vi "Generate Non Text Layer(s).vi"(0 "Library Path":path, 5 "new picture":picture, 7 "VI Refnum in":refnum<vi>, 11 "error in":errorcluster) -> (4 "Layers":refnum<class "Layer.lvclass">[](array[class]), 6 "Icon Height":i16, 15 "error out":errorcluster)   [LabVIEW 2024, in "Text-Based VI Icon.lvlib"]
uses:
  <vilib>/LabVIEW Icon API/Set Text Icon/Text-Based VI Icon.lvlib
  <vilib>/LabVIEW Icon API/lv_icon/Classes/Layer/Layer.lvclass
  <vilib>/LabVIEW Icon API/lv_icon/Controls/Layer.ctl
  <vilib>/LabVIEW Icon API/Set Text Icon/User Visible Strings.vi
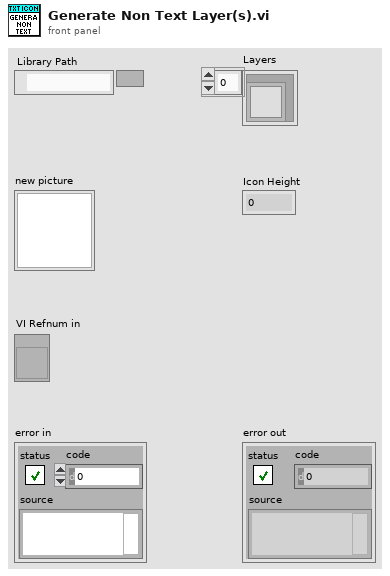
[diagram p1: front panel]
types:
  T1 = cluster{"left":i16, "top":i16, "right":i16, "bottom":i16}
  T2 = typedef "Layer.ctl" = cluster{"LayerIcon":picture, "LayerName":string, "Opacity":u8, "Visibility?":bool}
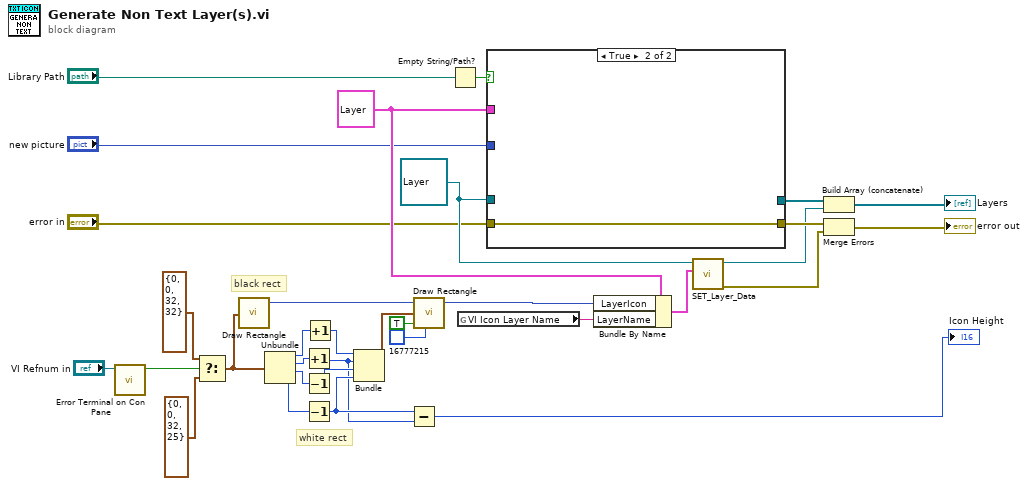
[diagram p0: block diagram]
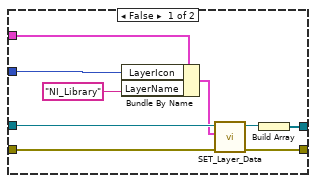
[diagram p2: hidden frame]
diagram:
  w21 = T2 {"LayerIcon"=bytes[3102], "LayerName"="", "Opacity"=100, "Visibility?"=TRUE} ("Data")
  w32 = refnum<class "Layer.lvclass"> refnum ("Layer.lvclass in")
  # "black rect"
  # "white rect"
  n1 = call <resource>:"Error Terminal on Con Pane.vi"("VI in"="VI Refnum in") -> ("Error Terminal on Con Pane?"=w11:bool)  [unwired: 9 in, 1 out]
  n2 = Select(t=T1 {"left"=0, "top"=0, "right"=32, "bottom"=32} ("rect"), s=w11, f=T1 {"left"=0, "top"=0, "right"=32, "bottom"=25} ("rect")) -> (s? t:f=w20:T1)
  n3 = call <vilib>:"Draw Rectangle.vi"("rect"=w20) -> ("new picture"=w31:picture)  [unwired: 8 in]
  n4 = Unbundle(w20) -> ("left"=w19:i16, "top"=w18:i16, "right"=w17:i16, "bottom"=w10:i16)
  n5 = Increment(x=w18) -> (x+1=w8:i16)
  n6 = Decrement(x=w17) -> (x-1=w15:i16)
  n7 = Decrement(x=w10) -> (x-1=w9:i16)
  n8 = Increment(x=w19) -> (x+1=w16:i16)
  n9 = Bundle(w16, w8, w15, w9) -> (w14:cluster{i16, i16, i16, i16})  [unwired: 1 in]
  n10 = Subtract(x=w9, y=w8) -> (x-y=→"Icon Height":i16)
  n11 = call <vilib>:"Draw Rectangle.vi"("picture"=w31, "rect"=w14, "fill?(F)"=TRUE, "color(black)"=u32 16777215) -> ("new picture"=w30:picture)  [unwired: 5 in]
  n12 = Empty String/Path?(string/path="Library Path") -> (empty?=w33:bool)
  n13 = global read "User Visible Strings.vi" "VI Icon Layer Name"() -> (w26:string)
  n14 = case shown="True" w33 {
    tunnel: "error in" -> [w40 w43]
    tunnel: w32 -> [w42 _]
    tunnel: w21 -> [w41 _]
    tunnel: [w36 w43] -> w25
    tunnel: [w35 _] -> w23
    tunnel: "new picture" -> [w34 _]
    frame False {
      n15 = Bundle By Name(cluster=w41, "LayerIcon"=w34, "LayerName"="NI_Library") -> (w39:T2)
      n16 = call-dynamic "SET_Layer_Data.vi"("error in (no error)"=w40, "Data"=w39, "Layer.lvclass in"=w42) -> ("error out"=w36:errorcluster, "Layer.lvclass out"=w37:refnum<class "Layer.lvclass">)  [unwired: 7 in]
      n17 = Build Array(w37) -> (w35:refnum<class "Layer.lvclass">[])
    }
    frame True {
    }
  }
  n18 = Bundle By Name(cluster=w21, "LayerIcon"=w30, "LayerName"=w26) -> (w27:T2)
  n19 = call-dynamic "SET_Layer_Data.vi"("Data"=w27, "Layer.lvclass in"=w32) -> ("error out"=w24:errorcluster, "Layer.lvclass out"=w22:refnum<class "Layer.lvclass">)  [unwired: 8 in]
  n20 = Build Array (concatenate)(w23, w22) -> (→"Layers":refnum<class "Layer.lvclass">[])
  n21 = Merge Errors(w25, w24) -> (→"error out":errorcluster)
